vi "Drive Controller.vi"(8 "error in":errorcluster) -> ()   [LabVIEW 2017]
doc: "This VI executes continuously carrying out the current operation and responding to updates or new operation requests. It will often contain the timing or control code that is difficult to place directly in TeleOp. This VI generally opens all sensors and motors and isolates the rest of the robot code from knowing implementation details of how the operations are carried out."
uses:
  <vilib>/Rock Robotics/WPI/Framework/Completion Status.ctl
  Drive Setpoints.ctl
  Drive Operations.ctl
  <vilib>/Rock Robotics/WPI/SafetyOutput/WPI_SafetyOutputConfigMenu.ctl
  <vilib>/Rock Robotics/SystemInterfaces/DIO/FPGA_DIOChannel.ctl
  <vilib>/Rock Robotics/WPI/RobotDrive/WPI_RobotDriveOpen2MotorWithTalon.vi
  <vilib>/Rock Robotics/WPI/Counter/WPI_CounterDigitalInputToDigitalSource.vi
panel:
  in  "Interactive Values":T1
  in  "Buttons":cluster{"Execute Cmd":bool, "Abort Cmd":bool}
  out "Command Timing":cluster{"Start Time (ms)":u32, "Iterations":i32}
  out "Status":T3
  out "Setpoints":T4(graph)
  out "Current\nCmd":string
  # "Tip: The graph shows the motor setpoints. It may also be helpful to observe inputs and sensor values.\nYou may also want to display tuning or debugging controls."
  # "Interactive Command: You may fill in the settings for a command\nand schedule it with the Execute button. You can observe and abort\nany command while fine tuning the code for the controller."
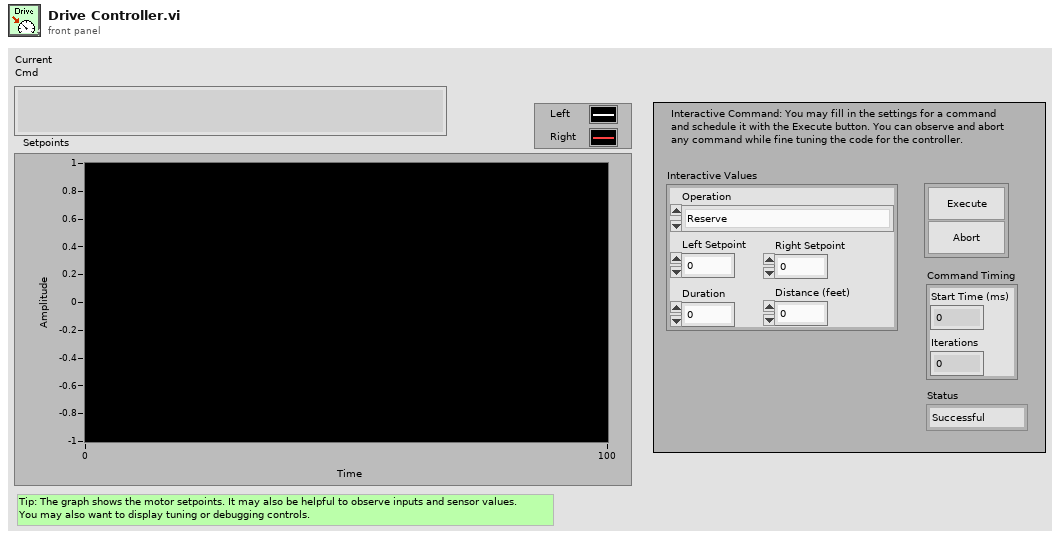
[diagram p1: front panel]
types:
  T1 = typedef "Drive Setpoints.ctl" = cluster{"Operation":T2, "Left Setpoint":dbl, "Right Setpoint":dbl, "Duration":dbl, "Distance (feet)":dbl}
  T2 = typedef "Drive Operations.ctl" = enum16{"Reserve", "Read Current", "Immediate", "Drive for Time", "Drive for Distance"}
  T3 = typedef "Completion Status.ctl" = enum16{"Successful", "Aborted", "Incomplete"}
  T4 = cluster{"Left Setpoint":dbl, "Right Setpoint":dbl}
  T5 = typedef "FPGA_DIOChannel.ctl" = enum8{"DIO 0", "DIO 1", "DIO 2", "DIO 3", "DIO 4", "DIO 5", "DIO 6", "DIO 7", "DIO 8", "DIO 9", "DIO MXP 0", "DIO MXP 1", "DIO MXP 2", "DIO MXP 3", "DIO MXP 4", "DIO MXP 5", "DIO MXP 6", "DIO MXP 7", "DIO MXP 8", "DIO MXP 9", "DIO MXP 10", "DIO MXP 11", "DIO MXP 12", "DIO MXP 13", "DIO MXP 14", "DIO MXP 15", "SPI Port CS1", "SPI Port CS2", "SPI Port CS3", "SPI Port MISO", "SPI Port MOSI", "Invalid"}
  T6 = typedef "WPI_SafetyOutputConfigMenu.ctl" = enum16{"Enable", "Disable"}
  T7 = typedef "WPI_RobotDriveDevRef.ctl" = cluster{"DevStatus":errorcluster, "Motors[]":T8[], "Square Inputs":bool, "Max Output":dbl}
  T8 = typedef "WPI_MotorControlDeviceRef.ctl" = cluster{"DeviceStatus":errorcluster, "Type":T9, "PWM":cluster{"PWM Channel":T10, "DeadBand":T11}, "CAN":cluster{"Device Number":u8, "SetOutput VI Ref":variant, "GetOutput VI Ref":variant, "Enable VI Ref":variant, "Disable VI Ref":variant, "Data":variant}, "Invert":bool, "DIO PWM":cluster{"PWM \"Enable\" Channel":T10, "DIOChannel":T5, "PWM Rate":dbl}}
  T9 = typedef "WPI_MotorControlType.ctl" = enum16{"PWM", "CAN", "DIO PWM"}
  T10 = typedef "FPGA_DIOPWMChannel.ctl" = enum8{"PWM 0", "PWM 1", "PWM 2", "PWM 3", "PWM 4", "PWM 5", "PWM 6", "PWM 7", "PWM 8", "PWM 9", "PWM MXP 0", "PWM MXP 1", "PWM MXP 2", "PWM MXP 3", "PWM MXP 4", "PWM MXP 5", "PWM MXP 6", "PWM MXP 7", "PWM MXP 8", "PWM MXP 9", "Invalid"}
  T11 = typedef "WPI_PWMDeadband.ctl" = cluster{"Name":string, "maxPositivePwm":i32, "minPositivePwm":i32, "centerPwm":i32, "maxNegativePwm":i32, "minNegativePwm":i32, "angularRange":u16}
  T12 = typedef "WPI_DigitalInputDevRef.ctl" = cluster{"DevStatus":errorcluster, "DIO Channel":T5}
  T13 = typedef "FPGA_CounterEncoderSourceConvertionLVSourceType.ctl" = cluster{"DevStatus":errorcluster, "AnalogTriggerMode?":bool, "DigitalMode":cluster{"DIO Channel":T14}, "AnalogTriggerMode":cluster{"AnalogTriggerIndex":T15, "OutputType":T16}}
  T14 = typedef "FPGA_DIODigitalSourceChannel.ctl" = enum8{"DIO 0", "DIO 1", "DIO 2", "DIO 3", "DIO 4", "DIO 5", "DIO 6", "DIO 7", "DIO 8", "DIO 9", "DIO MXP 0", "DIO MXP 1", "DIO MXP 2", "DIO MXP 3", "DIO MXP 4", "DIO MXP 5", "DIO MXP 6", "DIO MXP 7", "DIO MXP 8", "DIO MXP 9", "DIO MXP 10", "DIO MXP 11", "DIO MXP 12", "DIO MXP 13", "DIO MXP 14", "DIO MXP 15", "Disabled"}
  T15 = typedef "FPGA_AnalogTriggerIndex.ctl" = enum8{"Trig 0", "Trig 1", "Trig 2", "Trig 3", "Trig 4", "Trig 5", "Trig 6", "Trig 7", "Invalid"}
  T16 = typedef "FPGA_AnalogTriggerOutType.ctl" = enum16{"InWindow", "TriggerState", "Rising", "Falling"}
  T17 = typedef "WPI_EncoderDevRef.ctl" = cluster{"DevStatus":errorcluster, "EncoderIndex":T18, "CounterIndex":T19, "DistancePerCount":dbl, "Decoding Type":T20}
  T18 = typedef "FPGA_EncoderIdx.ctl" = enum8{"Enc 0", "Enc 1", "Enc 2", "Enc 3", "Enc 4", "Enc 5", "Enc 6", "Enc 7", "Invalid"}
  T19 = typedef "FPGA_CounterCtrSystemIndex.ctl" = enum8{"Ctr 0", "Ctr 1", "Ctr 2", "Ctr 3", "Ctr 4", "Ctr 5", "Ctr 6", "Ctr 7", "Invalid"}
  T20 = typedef "WPI_EncoderType.ctl" = enum16{"1x", "2x", "4x"}
  T21 = typedef "Command Status Info.ctl" = cluster{"Name":string, "Status":T3, "notifier out":T22}
  T22 = typedef "Completion Notifier.ctl" = refnum<notifier>
  T23 = cluster{"SubSystem Data":T1, cluster{"Start Time (ms)":u32, "Iterations":i32}, cluster{"Command Info":T21, "Description":string, "Default Command":T1, "queue out":refnum<queue>, "Subsystem Name":string}}
  T24 = cluster{"SubSystem Data":T1, cluster{"Start Time (ms)":u32, "Iterations":i32}, "Default Command Arguments":cluster{"Command Info":T21, "Description":string, "Default Command":T1, "queue out":refnum<queue>, "Subsystem Name":string}}
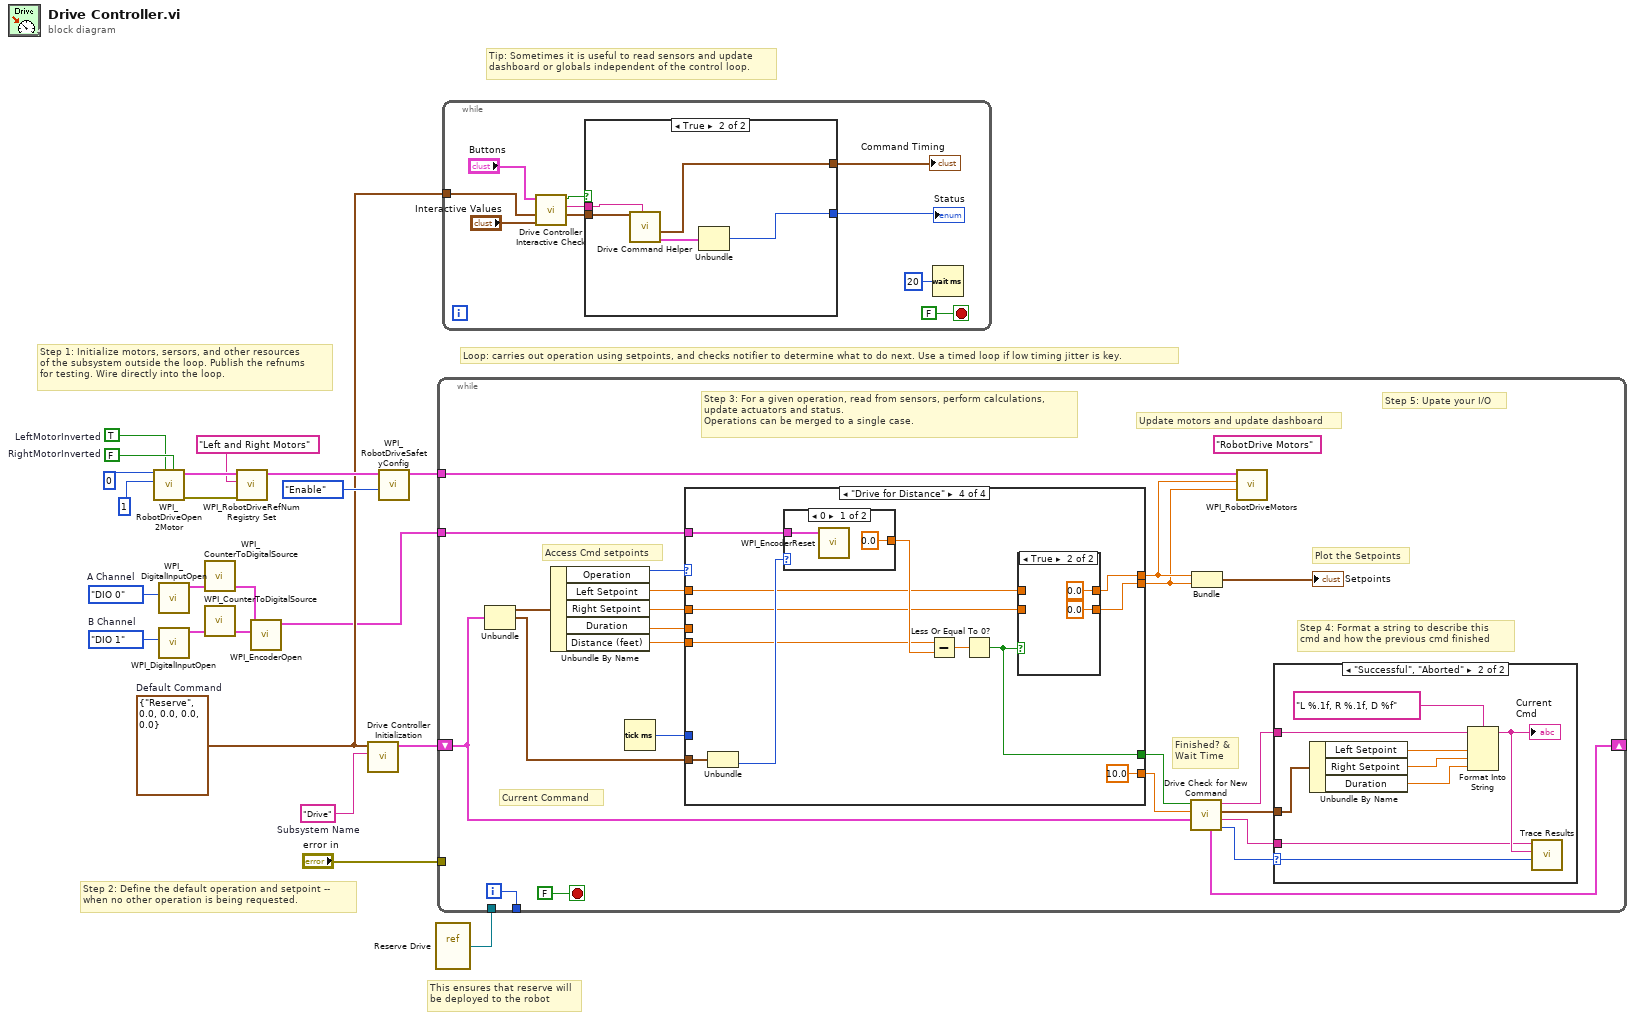
[diagram p0: block diagram]
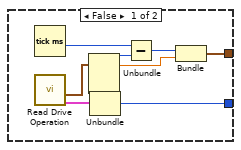
[diagram p2: hidden frame]
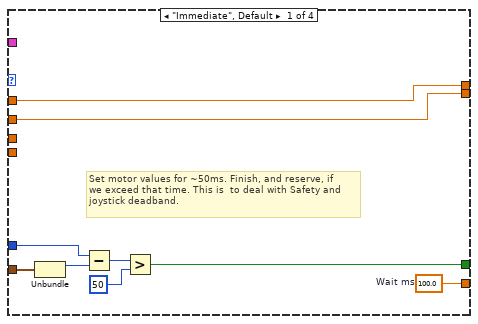
[diagram p4: hidden frame]
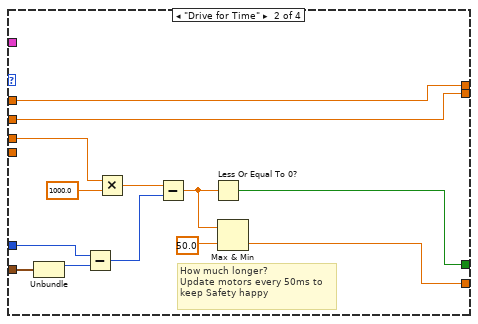
[diagram p5: hidden frame]
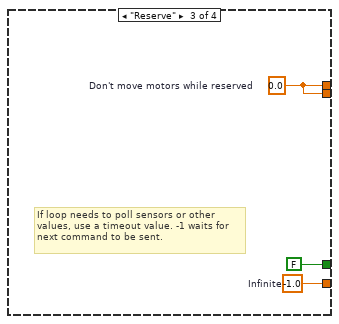
[diagram p6: hidden frame]
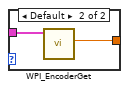
[diagram p8: hidden frame]
diagram:
  w7 = FPGA_DIOChannel."DIO 1"  # B Channel
  w6 = FPGA_DIOChannel."DIO 0"  # A Channel
  w18 = TRUE  # LeftMotorInverted
  w19 = FALSE  # RightMotorInverted
  w8 = T1 {"Operation"=enum."Reserve", "Left Setpoint"=0.0, "Right Setpoint"=0.0, "Duration"=0.0, "Distance (feet)"=0.0}  # Default Command
  w22 = "Drive"  # Subsystem Name
  # "This ensures that reserve will\nbe deployed to the robot"
  # "Tip: Sometimes it is useful to read sensors and update\ndashboard or globals independent of the control loop."
  # "Step 2: Define the default operation and setpoint --\nwhen no other operation is being requested."
  # "Step 1: Initialize motors, sersors, and other resources\nof the subsystem outside the loop. Publish the refnums\nfor testing. Wire directly into the loop."
  # "Loop: carries out operation using setpoints, and checks notifier to determine what to do next. Use a timed loop if low timing jitter is key."
  n1 = call-poly <vilib>:"WPI_RobotDriveOpen2Motor.vi"("Right Motor Inverted"=w19, "Left Motor Inverted"=w18, "Right Motor"=u8 1 ("Left Motor"), "Left Motor"=u8 0) -> ("error out"=w15:errorcluster, "RobotDriveDevRef"=w17:T7)  [unwired: 1 in, 5 out]
  n2 = call <vilib>:"WPI_DigitalInputOpen.vi"("DIO Channel"=w6) -> ("DigitalInputDevRef"=w3:T12)  [unwired: 1 in, 9 out]
  n3 = call <vilib>:"WPI_DigitalInputOpen.vi"("DIO Channel"=w7) -> ("DigitalInputDevRef"=w4:T12)  [unwired: 1 in, 9 out]
  n4 = call-poly <vilib>:"WPI_CounterToDigitalSource.vi"("DigitalInputDevRef"=w3) -> ("Digital Source"=w2:T13)  [unwired: 6 out]
  n5 = call-poly <vilib>:"WPI_CounterToDigitalSource.vi"("DigitalInputDevRef"=w4) -> ("Digital Source"=w5:T13)  [unwired: 6 out]
  n6 = call <vilib>:"WPI_RobotDriveRefNum Registry Set.vi"("error in (no error)"=w15, "refnum name"="Left and Right Motors", "RobotDriveDevRef"=w17) -> ("RobotDriveDevRef"=w14:T7)  [unwired: 1 in, 7 out]
  n7 = call <vilib>:"WPI_EncoderOpen.vi"("BSource"=w5, "ASource"=w2) -> ("EncoderDevRef"=w1:T17)  [unwired: 6 in, 3 out]
  n8 = call "Drive Controller Initialization.vi"("Subsystem Name"=w22, "Default Command"=w8) -> ("Current Command"=w10:T23)  [unwired: 9 in]
  n9 = call <vilib>:"WPI_RobotDriveSafetyConfig.vi"("mode"=WPI_SafetyOutputConfigMenu."Enable", "RobotDriveDevRef"=w14) -> ("RobotDriveDevRef"=w12:T7)  [unwired: 8 in, 1 out]
  n10 = vi-ref "Reserve Drive.vi"() -> (w9:refnum<vi>)
  n11 = while {
    shift-right: [w32] -> _
    shift-left: w10 -> [w25]
    tunnel: [w44] -> _
    tunnel: w12 -> [w40]
    tunnel: "error in" -> [_]
    tunnel: w9 -> [_]
    tunnel: w1 -> [w24]
    i -> [w44]
    stop <- FALSE stop-if-true
    (unwired) "RobotDrive Motors" ("Name")
    # "Step 5: Upate your I/O"
    # "Step 4: Format a string to describe this\ncmd and how the previous cmd finished"
    # "Current Command"
    # "Update motors and update dashboard"
    # "Plot the Setpoints"
    # "Access Cmd setpoints"
    # "Finished? &\nWait Time"
    # "Step 3: For a given operation, read from sensors, perform calculations,\nupdate actuators and status.\nOperations can be merged to a single case."
    n12 = Unbundle(w25) -> ("SubSystem Data"=w39:T1, w26:cluster{"Start Time (ms)":u32, "Iterations":i32})  [unwired: 1 out]
    n13 = Unbundle By Name(w39) -> ("Operation"=w38:T2, "Left Setpoint"=w37:dbl, "Right Setpoint"=w36:dbl, "Duration"=w35:dbl, "Distance (feet)"=w23:dbl)
    n14 = Tick Count (ms)() -> (millisecond timer value=w34:u32)
    n15 = case shown="\"Drive for Distance\"" w38 {
      tunnel: [w63 w64 w79 10.0 ("Infinite")] -> w31
      tunnel: [w56 w71 FALSE ("ignore previous (F)") w85] -> w30
      tunnel: w26 -> [w55 w73 _ w90]
      tunnel: [w62 w70 w77 w82] -> w42
      tunnel: [w61 w69 w77 w80] -> w41
      tunnel: w37 -> [w62 w70 _ w83]
      tunnel: w36 -> [w61 w69 _ w81]
      tunnel: w35 -> [_ w68 _ _]
      tunnel: w34 -> [w57 w67 _ _]
      tunnel: w24 -> [_ _ _ w91]
      tunnel: w23 -> [_ _ _ w87]
      frame "Immediate", Default {
        w63 = 100.0  # Wait ms
        # "Set motor values for ~50ms. Finish, and reserve, if\nwe exceed that time. This is  to deal with Safety and\njoystick deadband."
        n16 = Unbundle(w55) -> ("Start Time (ms)"=w58:u32)  [unwired: 1 out]
        n17 = Subtract(x=w57, y=w58) -> (x-y=w59:u32)
        n18 = Greater?(x=w59, y=u8 50 ("Left Motor")) -> (0:w56:bool)
      }
      frame "Drive for Time" {
        # "How much longer?\nUpdate motors every 50ms to\nkeep Safety happy"
        n19 = Unbundle(w73) -> ("Start Time (ms)"=w72:u32)  [unwired: 1 out]
        n20 = Subtract(x=w67, y=w72) -> (x-y=w76:u32)
        n21 = Multiply(x=w68, y=1000.0) -> (x*y=w75:dbl)
        n22 = Subtract(x=w75, y=w76) -> (x-y=w66:dbl)
        n23 = Less Or Equal To 0?(x=w66) -> (x <= 0?=w71:bool)
        n24 = Max & Min(x=w66, y=50.0) -> (min(x,y)=w64:dbl)  [unwired: 1 out]
      }
      frame "Reserve" {
        w77 = 0.0  # Don't move motors while reserved
        w79 = -1.0  # Infinite
        # "If loop needs to poll sensors or other\nvalues, use a timeout value. -1 waits for\nnext command to be sent."
      }
      frame "Drive for Distance" {
        n25 = Unbundle(w90) -> ("Iterations"=w89:i32)  [unwired: 1 out]
        n26 = case shown="0" w89 {
          tunnel: w91 -> [w97 w99]
          tunnel: [0.0 ("Distance") w98] -> w88
          frame 0 {
            n27 = call <vilib>:"WPI_EncoderReset.vi"("EncoderDevRef"=w97) -> ()  [unwired: 9 in, 2 out]
          }
          frame Default {
            n28 = call <vilib>:"WPI_EncoderGet.vi"("EncoderDevRef"=w99) -> ("Distance"=w98:dbl)  [unwired: 5 in, 5 out]
          }
        }
        n29 = Subtract(x=w87, y=w88) -> (x-y=w86:dbl)
        n30 = Less Or Equal To 0?(x=w86) -> (x <= 0?=w85:bool)
        n31 = case shown="True" w85 {
          tunnel: [w93 0.0 ("Left Setpoint")] -> w82
          tunnel: w83 -> [w93 _]
          tunnel: [w92 0.0 ("Right Setpoint")] -> w80
          tunnel: w81 -> [w92 _]
          frame False {
          }
          frame True {
          }
        }
      }
    }
    n32 = call "Drive Check for New Command.vi"("input cluster"=w25, "Wait time (ms)"=w31, "Finished?"=w30) -> ("Completion"=w33:T3, "Subsystem Name"=w27:string, "Current Command"=w28:T1, "Initial Trace String"=w29:string, "Next Command"=w32:T24)  [unwired: 4 in]
    n33 = Bundle("Left Setpoint"=w42, "Right Setpoint"=w41) -> (→"Setpoints":T4)  [unwired: 1 in]
    n34 = call <vilib>:"WPI_RobotDriveMotors.vi"("RightSpeed"=w41, "LeftSpeed"=w42, "RobotDriveDevRef"=w40) -> ()  [unwired: 1 in, 8 out]
    n35 = case shown="\"Successful\", \"Aborted\"" w33 {
      selector: w33 -> [_ w54]
      tunnel: w29 -> [_ w49]
      tunnel: w28 -> [_ w50]
      tunnel: w27 -> [_ w46]
      frame "Incomplete", Default {
        # "Continuing current command"
      }
      frame "Successful", "Aborted" {
        # "Report and setup for next command"
        n36 = Unbundle By Name(w50) -> ("Left Setpoint"=w52:dbl, "Right Setpoint"=w53:dbl, "Duration"=w47:dbl)
        n37 = Format Into String(format string="L %.1f, R %.1f, D %f", initial string=w49, w52, w53, w47) -> (resulting string=w48:string)  [unwired: 1 in, 1 out]
        "Current\nCmd" <- w48
        n38 = call <vilib>:"Trace Results.vi"("Status of previous command"=w54, "Description"=w48, "Subsystem"=w46) -> ()  [unwired: 9 in]
      }
    }
  }
  n39 = while {
    tunnel: w8 -> [w101]
    stop <- FALSE stop-if-true
    n40 = call "Drive Controller Interactive Check.vi"("Interactive Command In"="Interactive Values", "Default Command"=w101, "Buttons"="Buttons") -> ("Interactive Command Out"=w103:T1, "Trace String"=w104:string, "Schedule"=w105:bool)  [unwired: 6 in]
    n41 = case shown="True" w105 {
      tunnel: [w114 w122] -> w106
      tunnel: [w113 w118] -> w107
      tunnel: w104 -> [_ w120]
      tunnel: w103 -> [_ w119]
      frame False {
        n42 = Tick Count (ms)() -> (millisecond timer value=w117:u32)
        n43 = call "Read Drive Operation.vi"() -> ("Command Info"=w111:T21, "SubSystem Data"=w110:T1)  [unwired: 9 in, 1 out]
        n44 = Unbundle(w110) -> ("Operation"=w115:T2, "Left Setpoint"=w112:dbl)  [unwired: 3 out]
        n45 = Unbundle(w111) -> ("Status"=w114:T3)  [unwired: 2 out]
        n46 = Subtract(x=w117, y=w115) -> (x-y=w116:u32)
        n47 = Bundle(w116, "Left Setpoint"=w112) -> (w113:cluster{u32, "Left Setpoint":dbl})  [unwired: 1 in]
      }
      frame True {
        n48 = call "Drive Command Helper.vi"("Description"=w120, "SubSystem Data"=w119) -> ("Command Info Out"=w121:T21, "Command Timing"=w118:cluster{"Start Time (ms)":u32, "Iterations":i32})  [unwired: 7 in, 1 out]
        n49 = Unbundle(w121) -> ("Status"=w122:T3)  [unwired: 2 out]
      }
    }
    "Status" <- w106
    "Command Timing" <- w107
    n50 = Wait (ms)(milliseconds to wait=u32 20) -> ()  [unwired: 1 out]
  }
